vi "SPCReadFIFO_HH.vi"() -> (2 "count":i32, 3 "error out":errorcluster, 4 "buffer":u32[](array[numeric]))   [LabVIEW 2009]
uses:
  hhlib.dll
panel:
  in  "error in (no error)":errorcluster
  out "FiFoOverrun":bool
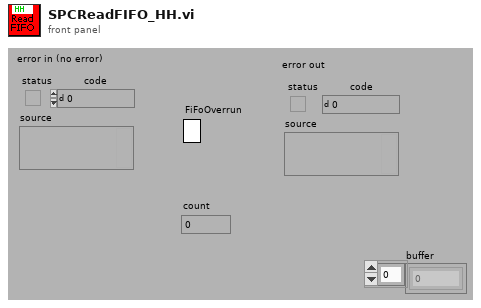
[diagram p1: front panel]
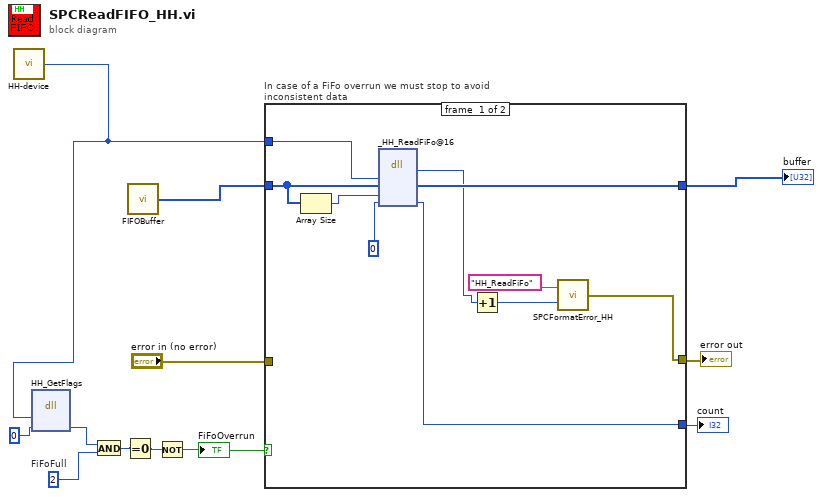
[diagram p0: block diagram]
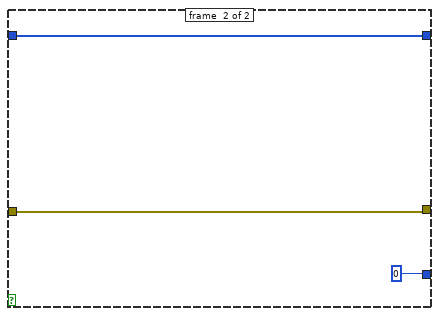
[diagram p2: hidden frame]
diagram:
  w9 = 2  # FiFoFull
  n1 = call "HH-device.vi"() -> ("Device (output)"=w1:i32)  [unwired: 2 in]
  n2 = dll-call lib="C:/Programme/Anwendungen/DAQLinescan_HH/hhlib.dll" fn="HH_GetFlags"("devidx"=w1, "flags"=0) -> ("flags"=w4:i32)  [unwired: 5 in, 2 out]
  n3 = And(x=w4, y=w9) -> (x .and. y?=w8:i32)
  n4 = Equal To 0?(x=w8) -> (x = 0?=w7:bool)
  n5 = call "FIFOBuffer.vi"() -> ("FIFOBuffer (output)"=w2:u32[])  [unwired: 2 in]
  n6 = Not ("CTCDone")(x=w7) -> (.not. x?=w6:bool)
  "FiFoOverrun" <- w6
  n7 = case "In case of a FiFo overrun we must stop to avoid inconsistent data" shown="False" w6 {
    tunnel: w2 -> [w16 w25]
    tunnel: [w19 0] -> w12
    tunnel: [w22 w25] -> w3
    tunnel: [w18 w24] -> w11
    tunnel: "error in (no error)" -> [_ w24]
    tunnel: w1 -> [w21 _]
    frame #0 {
      n8 = Array Size(array=w16) -> (size(s)=w15:i32)
      n9 = dll-call lib="C:/Programme/Anwendungen/DAQLinescan_HH/hhlib.dll" fn="_HH_ReadFiFo@16" label="HH_ReadFiFo"("devidx"=w21, "buffer"=w16, "blocksize"=w15, "nactual"=0) -> (w14:i32, "buffer"=w22:u32[], "nactual"=w19:i32)  [unwired: 5 in, 2 out]
      n10 = Increment(x=w14) -> (x+1=w13:i32)
      n11 = call "SPCFormatError_HH.vi"("Error Code"=w13, "Source"="HH_ReadFiFo") -> ("error out"=w18:errorcluster)
    }
    frame #1 {
    }
  }
  "count" <- w12
  "error out" <- w11
  "buffer" <- w3
